vi "Frame in Single Point.vi"() -> ()   [LabVIEW 2025]
uses:
  <vilib>/xnet/xnet.llb/XNET Frame CAN.ctl
  <vilib>/xnet/xnet.llb/XNET Frame Type CAN.ctl
  <vilib>/xnet/xnet.llb/XNET Create Session (Frame Input Single-point).vi
  <vilib>/xnet/xnet.llb/XNET Read (Frame CAN).vi
panel:
  out "data":T1[](array[typedef]) {"payload" format="%x"; "timestamp" format="%<%.7X\n%x>T"; "type" items=["CAN Data"=0, "CAN Remote"=1, "CAN Bus Error"=2, "CAN 2.0 Data"=8, "CAN FD Data"=16, "CAN FD+BRS Data"=24, "J1939 Data"=192, "Delay"=224, "Log Trigger"=225, "Start Trigger"=226]; "identifier" format="%x"}
  in  "Wait":u32=200
  in  "stop":bool
  in  "frame list":refnum<k21>[](array[refnum])=["Cardio\nSpartanGym"]
  in  "interface":refnum<k21>="CAN1"
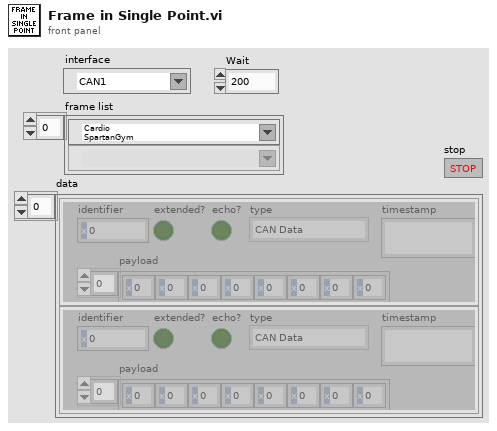
[diagram p1: front panel]
types:
  T1 = typedef "XNET Frame CAN.ctl" = cluster{"timestamp":timestamp, "payload":u8[], "identifier":u32, "type":T2, "extended?":bool, "echo?":bool}
  T2 = typedef "XNET Frame Type CAN.ctl" = u8
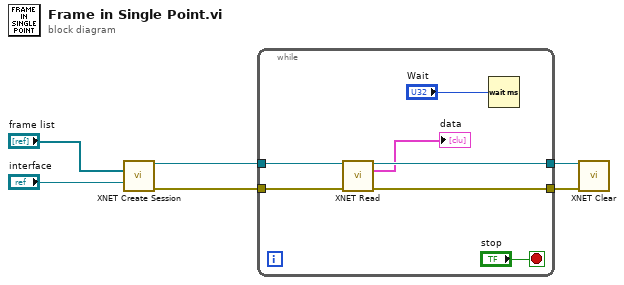
[diagram p0: block diagram]
diagram:
  n1 = call-poly <vilib>:"XNET Create Session.vi"("frame list"="frame list", "interface"="interface") -> ("session out"=w5:refnum<k21>, "error out"=w6:errorcluster)  [unwired: 12 in]
  n2 = while {
    tunnel: w6 -> [w12]
    tunnel: w5 -> [w13]
    tunnel: [w11] -> w2
    tunnel: [w10] -> w1
    stop <- "stop" stop-if-true
    n3 = call-poly <vilib>:"XNET Read.vi"("session in"=w13, "error in (no error)"=w12) -> ("session out"=w10:refnum<k21>, "data"=→"data":T1[], "error out"=w11:errorcluster)  [unwired: 10 in, 1 out]
    n4 = Wait (ms)(milliseconds to wait="Wait") -> ()  [unwired: 1 out]
  }
  n5 = call <vilib>:"XNET Clear.vi"("session in"=w1, "error in (no error)"=w2) -> ()  [unwired: 13 in, 1 out]
